vi "VITester.vi"() -> ()   [LabVIEW 2018]
panel:
  in  "Iterations":i32=50
  out "Sum_Total":dbl
  out "Total":dbl
  out "Total":dbl
  out "Total":dbl
  out "Free/CopyToCPU":dbl
  out "Open/Close":dbl
  out "Erode/Dilate":dbl
  out "Thres/Reverse":dbl
  out "Save/CopyToGPU":dbl
  in  "Blocks 1D":i32=640
  in  "Threads 1D":i32=1024
  in  "Partes / TODO Inicio":enum16{"Partes", "TODO"}(ring)=enum."TODO"
  in  "Open / Close":T1(ring)=enum."Nothing"
  in  "Partes / TODO Final":enum16{"Partes", "TODO"}(ring)=enum."TODO"
  in  "Erode / Dilate":T2(ring)=enum."Nothing"
  in  "Threshold / Reverse":T3(ring)=enum."Nothing"
  in  "ACQ / BMP":enum16{"Acq", "BMP"}(ring)
  out "Error OUT Toolkit":i32
  in  "Frame":u32=400
  in  "Threads 2D":i32=32
  in  "Blocks 2D":i32=1000
  in  "Radio":i32=1
  in  "max":u8=240
  in  "min":u8=70
  in  "IMAGE FILE PATH":path=path "C:/Users/AUTIS/Desktop/LibreriaAUTIS/Imagenes/IMG_BMP/Img_Or_Resampled[FRAME0271].bmp"
  in  "ACQ FILE PATH":path=path "C:/Users/AUTIS/Desktop/LibreriaAUTIS/Imagenes/IMG_BINARIA/[20190326][182154][654835][MONDEO_WGN][MAGNETIC][CAMERA21].acq"
  out "Error Out":errorcluster
  in  "Buffer Dst":string="BufferDst_Prueba"
  in  "Buffer Src":string="BufferSrc_Prueba"
  in  "Error In":errorcluster
  out "Image  Dst":T4(plugin-control)
  out "Image Src":T4(plugin-control)
  out "Nº Frames Facts":i32
  out "Total":dbl
  out "Total":dbl
  # "FILE'S PATH"
  # "Select nº Iterations"
  # "Threshold Values"
  # "Threshold Values"
  # "Other Algorithms"
  # "RADIO DE ERODE / DILATE"
  # "Select File To Process"
  # "Error OUT Toolkit"
  # "Src Image Buffer Name & Dst Image Buffer Name"
  # "Select Init ACQ\nFrame"
  # "Select type process"
  # "Time in ms"
  # "Total time in ms"
  # "Error IN / OUT LabVIEW"
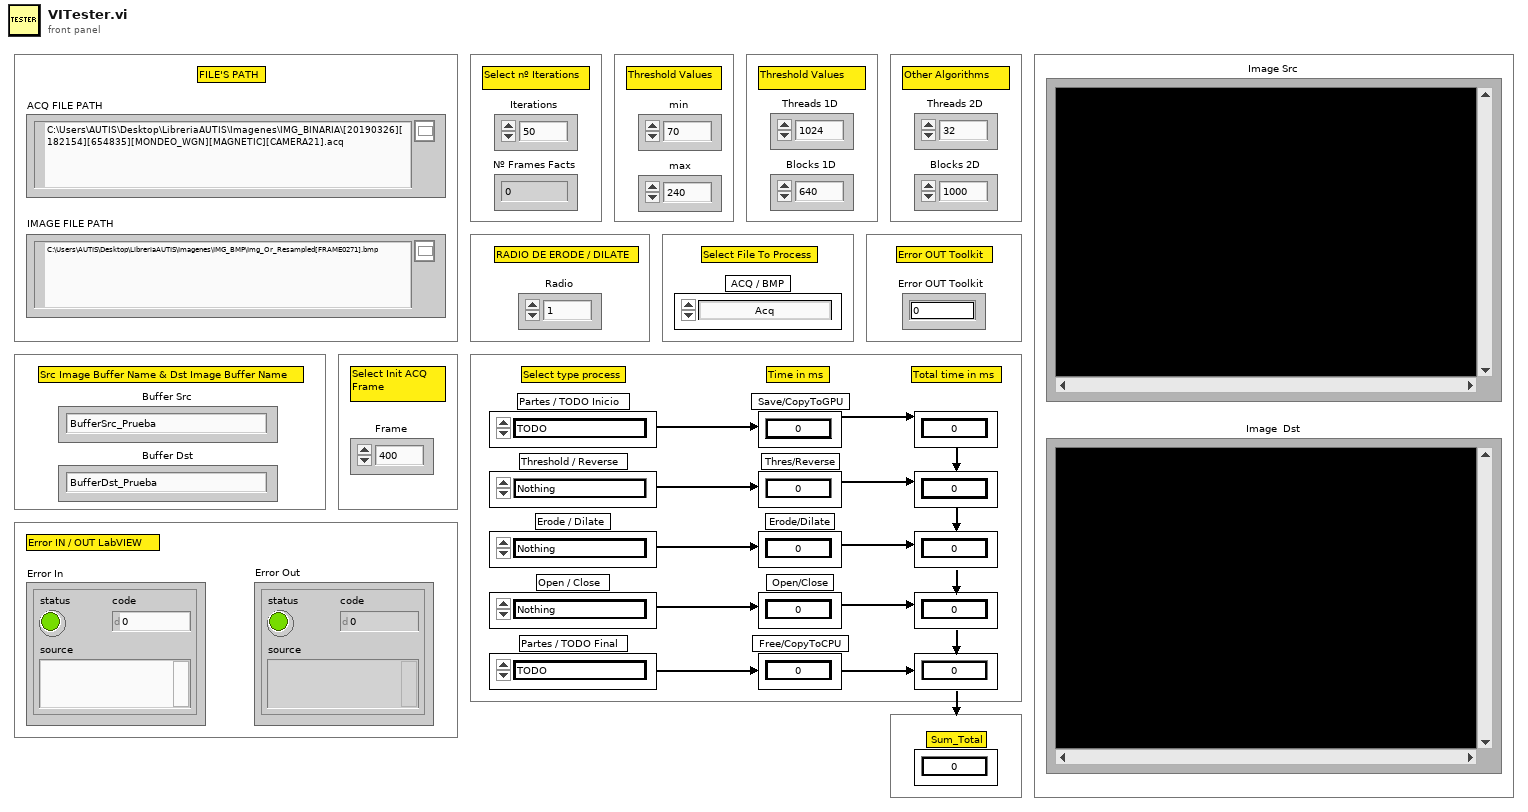
[diagram p1: front panel]
types:
  T1 = enum16{"Open_Fast_Auto", "Open_Fast_Manual", "Close_Fast_Auto", "Close_Fast_Manual", "Nothing"}
  T2 = enum16{"Erode_Low_Automatic", "Erode_Low_Manual", "Erode_Fast_Automatic", "Erode_Fast_Manual", "Dilate_Low_Automatic", "Dilate_Low_Manual", "Dilate_Fast_Automatic", "Dilate_Fast_Manual", "Nothing"}
  T3 = enum16{"Thres_Auto", "Thres_Manual", "Rev_Thres_Auto", "Rev_Thres_Manual", "Nothing"}
  T4 = typedef "IMAQ Image.ctl" = refnum<image>
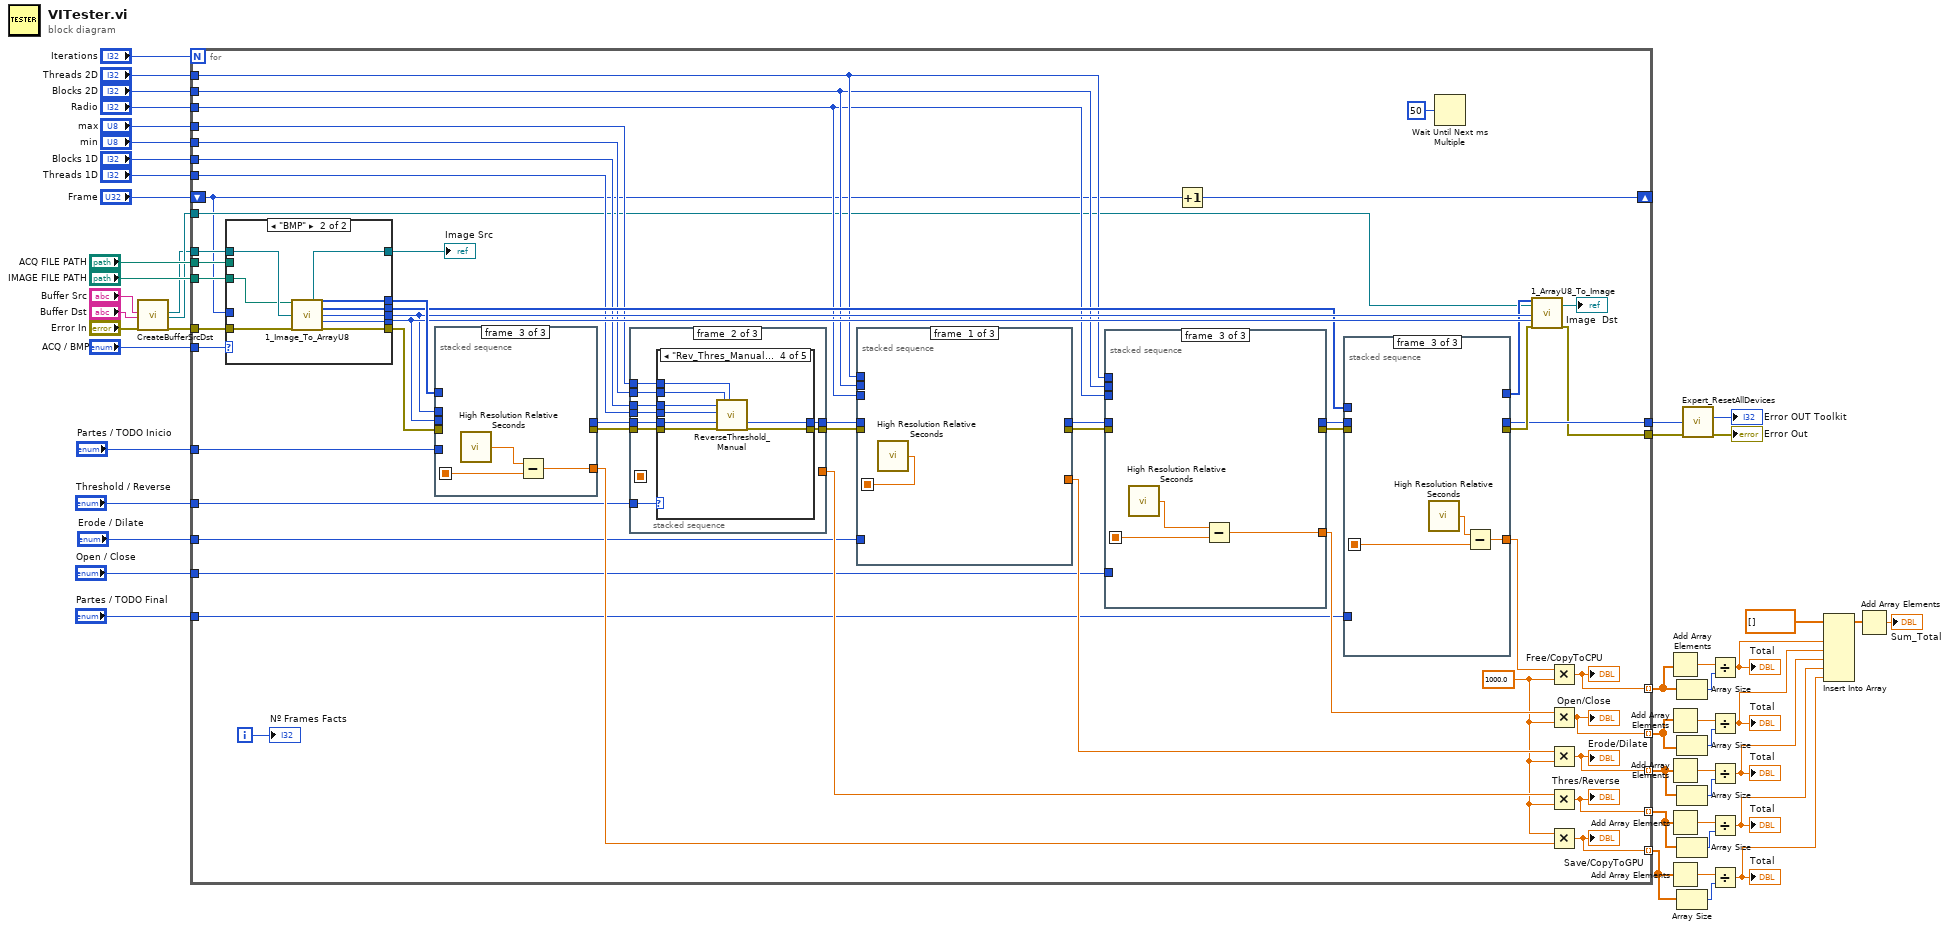
[diagram p0: block diagram]
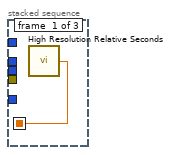
[diagram p2: hidden frame]
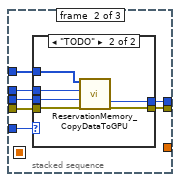
[diagram p3: hidden frame]
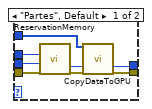
[diagram p4: hidden frame]
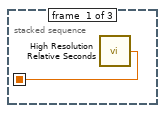
[diagram p5: hidden frame]
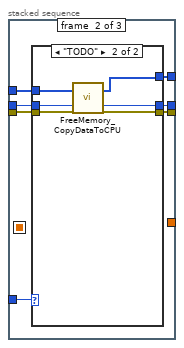
[diagram p6: hidden frame]
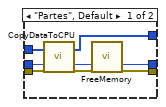
[diagram p7: hidden frame]
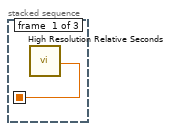
[diagram p8: hidden frame]
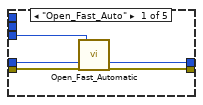
[diagram p10: hidden frame]
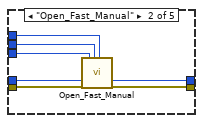
[diagram p11: hidden frame]
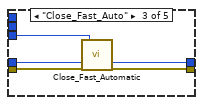
[diagram p12: hidden frame]
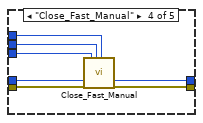
[diagram p13: hidden frame]
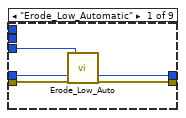
[diagram p15: hidden frame]
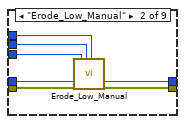
[diagram p16: hidden frame]
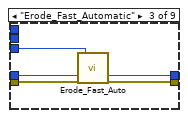
[diagram p17: hidden frame]
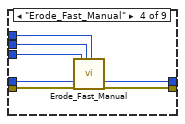
[diagram p18: hidden frame]
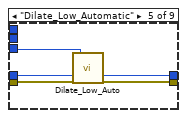
[diagram p19: hidden frame]
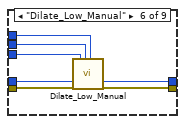
[diagram p20: hidden frame]
diagram:
  n1 = call "CreateBufferSrcDst.vi"("Buffer Src Name"="Buffer Src", "Buffer Dst Name"="Buffer Dst", "Error IN"="Error In") -> ("Image Src Result"=w14:T4, "Image Dst Result"=w15:T4, "Error OUT"=w16:errorcluster)  [unwired: 14 in]
  n2 = for {
    N: "Iterations" -> [_]
    tunnel: "Blocks 1D" -> [w80]
    tunnel: "Threads 1D" -> [w79]
    tunnel: "Partes / TODO Inicio" -> [w78]
    tunnel: "Open / Close" -> [w77]
    tunnel: "Partes / TODO Final" -> [w76]
    tunnel: "Erode / Dilate" -> [w75]
    tunnel: "Threshold / Reverse" -> [w74]
    tunnel: "ACQ / BMP" -> [w73]
    tunnel: "Threads 2D" -> [w72]
    tunnel: "Blocks 2D" -> [w71]
    tunnel: "Radio" -> [w66]
    tunnel: "max" -> [w70]
    tunnel: "min" -> [w69]
    tunnel: "IMAGE FILE PATH" -> [w68]
    tunnel: "ACQ FILE PATH" -> [w67]
    tunnel: [w65] -> w22 mode=indexing
    tunnel: [w64] -> w21 mode=indexing
    tunnel: [w63] -> w24 mode=indexing
    tunnel: [w62] -> w23 mode=indexing
    tunnel: [w61] -> w20 mode=indexing
    tunnel: w16 -> [w58]
    shift-right: [w51] -> _
    shift-left: "Frame" -> [w54]
    tunnel: w15 -> [w56]
    tunnel: w14 -> [w55]
    tunnel: [w53] -> w5
    tunnel: [w52] -> w4
    i -> [w102]
    w81 = 1000.0 ("y")
    n3 = case shown="\"BMP\"" w73 {
      tunnel: w58 -> [w305 w315]
      tunnel: w55 -> [w302 w314]
      tunnel: [w299 w313] -> w57
      tunnel: [w301 w312] -> w99
      tunnel: [w303 w311] -> w89
      tunnel: w67 -> [w306 _]
      tunnel: w68 -> [_ w310]
      tunnel: w54 -> [w304 _]
      tunnel: [w298 w309] -> w100
      tunnel: [w297 w308] -> w98
      tunnel: [w296 w307] -> w97
      frame "Acq", Default {
        n4 = call "1_acq_To_ArrayU8.vi"("File path"=w306, "Frame"=w304, "error in"=w305) -> ("Array Src OUT"=w301:u8[], "Array Dst OUT"=w303:u8[], "Width"=w296:i32, "Height"=w297:i32, "Error Out"=w300:errorcluster)  [unwired: 12 in]
        n5 = call "1_ArrayU8_To_Image.vi"("Array Src IN"=w301, "Buffer Image"=w302, "Width"=w296, "Height"=w297, "Error in"=w300) -> ("Image"=w299:T4, "Error out"=w298:errorcluster)  [unwired: 13 in]
      }
      frame "BMP" {
        n6 = call "1_Image_To_ArrayU8.vi"("Image Path"=w310, "Buffer Src IN"=w314, "Error IN"=w315) -> ("Image Src OUT"=w313:T4, "Array Src OUT"=w312:u8[], "Array Dst OUT"=w311:u8[], "Width or X"=w307:i32, "Height or Y"=w308:i32, "Error OUT"=w309:errorcluster)  [unwired: 7 in]
      }
    }
    "Image Src" <- w57
    n7 = stacked-sequence {
      seq-local: [w103 _ _] -> [_ _ w125]
      tunnel: [_ _ w127] -> w86
      tunnel: w78 -> [_ w110 _]
      tunnel: w100 -> [_ w109 _]
      tunnel: w97 -> [_ w108 _]
      tunnel: w99 -> [_ w107 _]
      tunnel: w98 -> [_ w106 _]
      tunnel: [_ w105 _] -> w96
      tunnel: [_ w104 _] -> w95
      frame #0 {
        n8 = call <vilib>:"High Resolution Relative Seconds.vi"() -> ("relative seconds"=w103:dbl)
      }
      frame #1 {
        n9 = case shown="\"TODO\"" w110 {
          tunnel: w109 -> [w116 w121]
          tunnel: w106 -> [w115 w122]
          tunnel: w108 -> [w114 w123]
          tunnel: w107 -> [w111 w124]
          tunnel: [w113 w120] -> w105
          tunnel: [w112 w119] -> w104
          frame "Partes", Default {
            n10 = call "ReservationMemory.vi"("Width"=w114, "Height"=w115, "Error IN LabVIEW"=w116) -> ("Error OUT Toolkit"=w118:i32, "Error OUT LabVIEW"=w117:errorcluster)  [unwired: 15 in]
            n11 = call "CopyDataToGPU.vi"("Array Src IN Host"=w111, "Error IN Toolkit"=w118, "Error IN LabVIEW"=w117) -> (18:"Error OUT LabVIEW"=w112:i32, 19:"Error OUT LabVIEW"=w113:errorcluster)  [unwired: 15 in]
          }
          frame "TODO" {
            n12 = call "ReservationMemory_CopyDataToGPU.vi"("Array Src In Host"=w124, "Width"=w123, "Height"=w122, "Error In LabVIEW"=w121) -> ("Error OUT Toolkit"=w119:i32, "Error Out LabVIEW"=w120:errorcluster)  [unwired: 14 in]
          }
        }
      }
      frame #2 {
        n13 = call <vilib>:"High Resolution Relative Seconds.vi"() -> ("relative seconds"=w126:dbl)
        n14 = Subtract(x=w126, y=w125) -> (x-y=w127:dbl)
      }
    }
    n15 = stacked-sequence {
      seq-local: [w253 _ _] -> [_ _ w293]
      tunnel: [_ _ w295] -> w85
      tunnel: w74 -> [_ w262 _]
      tunnel: w96 -> [_ w261 _]
      tunnel: w95 -> [_ w260 _]
      tunnel: [_ w259 _] -> w60
      tunnel: [_ w258 _] -> w94
      tunnel: w69 -> [_ w257 _]
      tunnel: w70 -> [_ w256 _]
      tunnel: w79 -> [_ w255 _]
      tunnel: w80 -> [_ w254 _]
      frame #0 {
        n16 = call <vilib>:"High Resolution Relative Seconds.vi"() -> ("relative seconds"=w253:dbl)
      }
      frame #1 {
        n17 = case shown="\"Rev_Thres_Manual\"" w262 {
          tunnel: [w267 w276 w281 w289 w292] -> w259
          tunnel: w261 -> [w268 w275 w282 w290 w292]
          tunnel: w260 -> [w265 w273 w279 w288 w291]
          tunnel: [w266 w274 w280 w283 w291] -> w258
          tunnel: w255 -> [_ w272 _ w287 _]
          tunnel: w254 -> [_ w271 _ w286 _]
          tunnel: w257 -> [w264 w270 w278 w285 _]
          tunnel: w256 -> [w263 w269 w277 w284 _]
          frame "Thres_Auto" {
            n18 = call "Threshold_Automatic.vi"("Error IN Toolkit"=w265, "Error IN LabVIEW"=w268, "min"=w264, "max"=w263) -> ("Error OUT Toolkit"=w266:i32, "Error OUT LabVIEW"=w267:errorcluster)  [unwired: 14 in]
          }
          frame "Thres_Manual" {
            n19 = call "Threshold_Manual.vi"("blocks"=w271, "threads"=w272, "Error IN Toolkit"=w273, "Error IN LabVIEW"=w275, "min"=w270, "max"=w269) -> ("Error OUT Toolkit"=w274:i32, "Error OUT LabVIEW"=w276:errorcluster)  [unwired: 12 in]
          }
          frame "Rev_Thres_Auto" {
            n20 = call "ReverseThreshold_Automatic.vi"("Error IN Toolkit"=w279, "Error IN LabVIEW"=w282, "min"=w278, "max"=w277) -> ("Error OUT Toolkit"=w280:i32, "Error OUT LabVIEW"=w281:errorcluster)  [unwired: 14 in]
          }
          frame "Rev_Thres_Manual" {
            n21 = call "ReverseThreshold_Manual.vi"("blocks"=w286, "threads"=w287, "Error IN Toolkit"=w288, "Error IN LabVIEW"=w290, "min"=w285, "max"=w284) -> ("Error OUT Toolkit"=w283:i32, "Error OUT LabVIEW"=w289:errorcluster)  [unwired: 12 in]
          }
          frame "Nothing", Default {
          }
        }
      }
      frame #2 {
        n22 = call <vilib>:"High Resolution Relative Seconds.vi"() -> ("relative seconds"=w294:dbl)
        n23 = Subtract(x=w294, y=w293) -> (x-y=w295:dbl)
      }
    }
    n24 = stacked-sequence {
      seq-local: [w191 _ _] -> [_ _ w250]
      tunnel: [_ _ w252] -> w84
      tunnel: w75 -> [_ w199 _]
      tunnel: w60 -> [_ w198 _]
      tunnel: w94 -> [_ w197 _]
      tunnel: w66 -> [_ w196 _]
      tunnel: w71 -> [_ w195 _]
      tunnel: w72 -> [_ w194 _]
      tunnel: [_ w193 _] -> w93
      tunnel: [_ w192 _] -> w92
      frame #0 {
        n25 = call <vilib>:"High Resolution Relative Seconds.vi"() -> ("relative seconds"=w191:dbl)
      }
      frame #1 {
        n26 = case shown="\"Nothing\", Default" w199 {
          tunnel: [w204 w211 w216 w223 w228 w235 w239 w247 w249] -> w193
          tunnel: [w203 w210 w215 w222 w225 w232 w238 w246 w248] -> w192
          tunnel: w195 -> [_ w209 _ w221 _ w234 _ w245 _]
          tunnel: w194 -> [_ w208 _ w220 _ w233 _ w244 _]
          tunnel: w198 -> [w202 w207 w214 w219 w227 w231 w240 w243 w249]
          tunnel: w197 -> [w201 w206 w213 w218 w226 w230 w237 w242 w248]
          tunnel: w196 -> [w200 w205 w212 w217 w224 w229 w236 w241 _]
          frame "Erode_Low_Automatic" {
            n27 = call "Erode_Low_Auto.vi"("Error IN Toolkit"=w201, "Error IN LabVIEW"=w202, "Radio"=w200) -> ("Error OUT Toolkit"=w203:i32, "Error OUT LabVIEW"=w204:errorcluster)  [unwired: 15 in]
          }
          frame "Erode_Low_Manual" {
            n28 = call "Erode_Low_Manual.vi"("Error IN Toolkit"=w206, "Error IN LabVIEW"=w207, "Radio"=w205, "Blocks"=w209, "Threads"=w208) -> ("Error OUT Toolkit"=w210:i32, "Error OUT LabVIEW"=w211:errorcluster)  [unwired: 13 in]
          }
          frame "Erode_Fast_Automatic" {
            n29 = call "Erode_Fast_Auto.vi"("Error IN Toolkit"=w213, "Error IN LabVIEW"=w214, "Radio"=w212) -> ("Error OUT Toolkit"=w215:i32, "Error OUT LabVIEW"=w216:errorcluster)  [unwired: 15 in]
          }
          frame "Erode_Fast_Manual" {
            n30 = call "Erode_Fast_Manual.vi"("Error IN Toolkit"=w218, "Error IN LabVIEW"=w219, "Radio"=w217, "Blocks"=w221, "Threads"=w220) -> ("Error OUT Toolkit"=w222:i32, "Error OUT LabVIEW"=w223:errorcluster)  [unwired: 13 in]
          }
          frame "Dilate_Low_Automatic" {
            n31 = call "Dilate_Low_Auto.vi"("Error IN Toolkit"=w226, "Error IN LabVIEW"=w227, "Radio"=w224) -> ("Error OUT Toolkit"=w225:i32, "Error OUT LabVIEW"=w228:errorcluster)  [unwired: 15 in]
          }
          frame "Dilate_Low_Manual" {
            n32 = call "Dilate_Low_Manual.vi"("Error IN Toolkit"=w230, "Error IN LabVIEW"=w231, "Radio"=w229, "Blocks"=w234, "Threads"=w233) -> ("Error OUT Toolkit"=w232:i32, "Error OUT LabVIEW"=w235:errorcluster)  [unwired: 13 in]
          }
          frame "Dilate_Fast_Automatic" {
            n33 = call "Dilate_Fast_Auto.vi"("Error IN Toolkit"=w237, "Error IN LabVIEW"=w240, "Radio"=w236) -> ("Error OUT Toolkit"=w238:i32, "Error OUT LabVIEW"=w239:errorcluster)  [unwired: 15 in]
          }
          frame "Dilate_Fast_Manual" {
            n34 = call "Dilate_Fast_Manual.vi"("Error IN Toolkit"=w242, "Error IN LabVIEW"=w243, "Radio"=w241, "Blocks"=w245, "Threads"=w244) -> ("Error OUT Toolkit"=w246:i32, "Error OUT LabVIEW"=w247:errorcluster)  [unwired: 13 in]
          }
          frame "Nothing", Default {
          }
        }
      }
      frame #2 {
        n35 = call <vilib>:"High Resolution Relative Seconds.vi"() -> ("relative seconds"=w251:dbl)
        n36 = Subtract(x=w251, y=w250) -> (x-y=w252:dbl)
      }
    }
    n37 = stacked-sequence {
      seq-local: [w153 _ _] -> [_ _ w188]
      tunnel: [_ _ w190] -> w82
      tunnel: w77 -> [_ w161 _]
      tunnel: w66 -> [_ w160 _]
      tunnel: w71 -> [_ w159 _]
      tunnel: w72 -> [_ w158 _]
      tunnel: w93 -> [_ w157 _]
      tunnel: w92 -> [_ w156 _]
      tunnel: [_ w155 _] -> w91
      tunnel: [_ w154 _] -> w90
      frame #0 {
        n38 = call <vilib>:"High Resolution Relative Seconds.vi"() -> ("relative seconds"=w153:dbl)
      }
      frame #1 {
        n39 = case shown="\"Nothing\", Default" w161 {
          tunnel: [w166 w173 w178 w185 w187] -> w155
          tunnel: [w165 w172 w177 w184 w186] -> w154
          tunnel: w160 -> [w164 w171 w176 w183 _]
          tunnel: w159 -> [_ w170 _ w182 _]
          tunnel: w158 -> [_ w169 _ w181 _]
          tunnel: w157 -> [w163 w168 w175 w180 w187]
          tunnel: w156 -> [w162 w167 w174 w179 w186]
          frame "Open_Fast_Auto" {
            n40 = call "Open_Fast_Automatic.vi"("Error IN Toolkit"=w162, "Error IN LabVIEW"=w163, "Radio"=w164) -> ("Error OUT Toolkit"=w165:i32, "Error OUT LabVIEW"=w166:errorcluster)  [unwired: 15 in]
          }
          frame "Open_Fast_Manual" {
            n41 = call "Open_Fast_Manual.vi"("Error IN Toolkit"=w167, "Error IN LabVIEW"=w168, "Radio"=w171, "blocks"=w170, "threads"=w169) -> ("Error OUT Toolkit"=w172:i32, "Error OUT LabVIEW"=w173:errorcluster)  [unwired: 13 in]
          }
          frame "Close_Fast_Auto" {
            n42 = call "Close_Fast_Automatic.vi"("Error IN Toolkit"=w174, "Error IN LabVIEW"=w175, "Radio"=w176) -> ("Error OUT Toolkit"=w177:i32, "Error OUT LabVIEW"=w178:errorcluster)  [unwired: 15 in]
          }
          frame "Close_Fast_Manual" {
            n43 = call "Close_Fast_Manual.vi"("Error IN Toolkit"=w179, "Error IN LabVIEW"=w180, "Radio"=w183, "Blocks"=w182, "Threads"=w181) -> ("Error OUT Toolkit"=w184:i32, "Error OUT LabVIEW"=w185:errorcluster)  [unwired: 13 in]
          }
          frame "Nothing", Default {
          }
        }
      }
      frame #2 {
        n44 = call <vilib>:"High Resolution Relative Seconds.vi"() -> ("relative seconds"=w189:dbl)
        n45 = Subtract(x=w189, y=w188) -> (x-y=w190:dbl)
      }
    }
    n46 = Increment(x=w54) -> (x+1=w51:u32)
    n47 = stacked-sequence {
      seq-local: [w128 _ _] -> [_ _ w150]
      tunnel: [_ _ w152] -> w83
      tunnel: w76 -> [_ w135 _]
      tunnel: w91 -> [_ w134 _]
      tunnel: w90 -> [_ w133 _]
      tunnel: w89 -> [_ w132 _]
      tunnel: [_ w131 _] -> w88
      tunnel: [_ w130 _] -> w87
      tunnel: [_ w129 _] -> w53
      frame #0 {
        n48 = call <vilib>:"High Resolution Relative Seconds.vi"() -> ("relative seconds"=w128:dbl)
      }
      frame #1 {
        n49 = case shown="\"TODO\"" w135 {
          tunnel: w134 -> [w141 w148]
          tunnel: w133 -> [w140 w147]
          tunnel: w132 -> [w139 w145]
          tunnel: [w138 w144] -> w131
          tunnel: [w137 w149] -> w130
          tunnel: [w136 w146] -> w129
          frame "Partes", Default {
            n50 = call "CopyDataToCPU.vi"("Array Dst IN Host"=w139, "Error IN Toolkit"=w140, "Error IN LabVIEW"=w141) -> ("Array Dst OUT Host"=w138:u8[], "Error OUT Toolkit"=w143:i32, "Error OUT LabVIEW"=w142:errorcluster)  [unwired: 14 in]
            n51 = call "FreeMemory.vi"("Error IN Toolkit"=w143, "Error IN LabVIEW"=w142) -> ("Error OUT Toolkit"=w136:i32, "Error OUT LabVIEW"=w137:errorcluster)  [unwired: 16 in]
          }
          frame "TODO" {
            n52 = call "FreeMemory_CopyDataToCPU.vi"("Array Dst In Host"=w145, "Error IN Toolkit"=w147, "Error In LabVIEW"=w148) -> ("Array Dst OUT Host"=w144:u8[], "Error OUT Toolkit"=w146:i32, "Error Out LabVIEW"=w149:errorcluster)  [unwired: 14 in]
          }
        }
      }
      frame #2 {
        n53 = call <vilib>:"High Resolution Relative Seconds.vi"() -> ("relative seconds"=w151:dbl)
        n54 = Subtract(x=w151, y=w150) -> (x-y=w152:dbl)
      }
    }
    n55 = Wait Until Next ms Multiple(millisecond multiple=u32 50) -> ()  [unwired: 1 out]
    n56 = call "1_ArrayU8_To_Image.vi"("Array Src IN"=w88, "Buffer Image"=w56, "Width"=w97, "Height"=w98, "Error in"=w87) -> ("Image"=→"Image  Dst":T4, "Error out"=w52:errorcluster)  [unwired: 13 in]
    n57 = Multiply(x=w83, y=w81) -> (x*y=w61:dbl)
    "Free/CopyToCPU" <- w61
    n58 = Multiply(x=w82, y=w81) -> (x*y=w62:dbl)
    "Open/Close" <- w62
    n59 = Multiply(x=w84, y=w81) -> (x*y=w63:dbl)
    "Erode/Dilate" <- w63
    n60 = Multiply(x=w85, y=w81) -> (x*y=w64:dbl)
    "Thres/Reverse" <- w64
    n61 = Multiply(x=w81, y=w86) -> (x*y=w65:dbl)
    "Save/CopyToGPU" <- w65
    "Nº Frames Facts" <- w102
  }
  n62 = Add Array Elements(numeric array=w20) -> (sum=w48:dbl)
  n63 = Add Array Elements(numeric array=w23) -> (sum=w31:dbl)
  n64 = Add Array Elements(numeric array=w24) -> (sum=w28:dbl)
  n65 = Add Array Elements(numeric array=w21) -> (sum=w27:dbl)
  n66 = Add Array Elements(numeric array=w22) -> (sum=w25:dbl)
  n67 = Array Size(array=w20) -> (size(s)=w49:i32)
  n68 = Array Size(array=w23) -> (size(s)=w30:i32)
  n69 = Array Size(array=w24) -> (size(s)=w29:i32)
  n70 = Array Size(array=w21) -> (size(s)=w26:i32)
  n71 = Array Size(array=w22) -> (size(s)=w47:i32)
  n72 = call "Expert_ResetAllDevices.vi"("Error IN Toolkit"=w5, "Error IN LabVIEW"=w4) -> ("Error OUT Toolkit"=→"Error OUT Toolkit":i32, "Error OUT LabVIEW"=→"Error Out":errorcluster)  [unwired: 12 in]
  n73 = Divide(x=w48, y=w49) -> (x/y=w13:dbl)
  "Total" <- w13
  n74 = Divide(x=w31, y=w30) -> (x/y=w12:dbl)
  "Total" <- w12
  n75 = Divide(x=w28, y=w29) -> (x/y=w11:dbl)
  "Total" <- w11
  n76 = Divide(x=w27, y=w26) -> (x/y=w10:dbl)
  "Total" <- w10
  n77 = Divide(x=w25, y=w47) -> (x/y=w9:dbl)
  "Total" <- w9
  n78 = Insert Into Array(array=dbl[] [], new element #1=w13, new element #2=w12, new element #3=w11, new element #4=w10, new element #5=w9) -> (w8:dbl[])  [unwired: 1 in]
  n79 = Add Array Elements(numeric array=w8) -> (sum=→"Sum_Total":dbl)
